vi "DAQ.Write.vi"(8 "error in (no error)":errorcluster, 10 "Write":T1, 11 "DAQmx.AO in":refnum<class "DAQmx.AO.lvclass">) -> (0 "error out":errorcluster, 2 "Written Waveform":waveform(dbl)[](array[waveform]), 3 "DAQmx.AO out":refnum<class "DAQmx.AO.lvclass">)   [LabVIEW 2016, in "DAQmx.AO.lvclass"]
uses:
  DAQmx.AO.lvclass
  C:/user/patrick/hg/levy_inst_lockin/src/SMOs/DAQmx/DAQmx.lvclass
  DAQ/Typedefs/PrivateEvents--DAQ.Write.ctl
  DAQmx/DAQmx.lvclass/DAQmx.ctl
  <vilib>/DAQmx/write.llb/DAQmx Write (Analog 1D Wfm NChan NSamp).vi
  <vilib>/DAQmx/miscellaneous.llb/DAQmx Fill In Error Info.vi
  <resource>/objmgr/daqmx.rc
  DAQmx/DAQmx.lvclass
  DAQ/DAQ.lvclass
panel:
  out "number of samples written per channel":u32
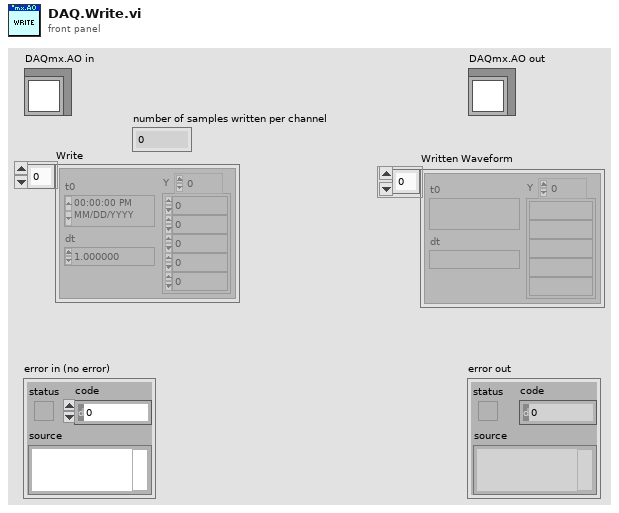
[diagram p1: front panel]
types:
  T1 = typedef "DAQ.lvclass/PrivateEvents--DAQ.Write.ctl" = waveform(dbl)[]
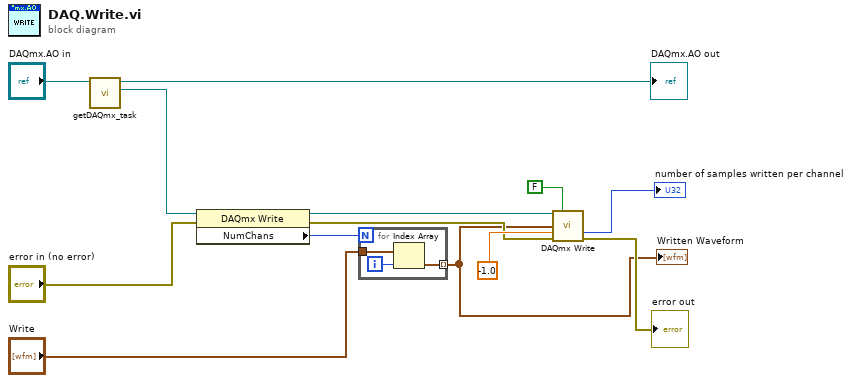
[diagram p0: block diagram]
diagram:
  n1 = call "getDAQmx_task.vi"("DAQmx in"="DAQmx.AO in") -> ("task"=w8:refnum<k21>, "DAQmx out"=→"DAQmx.AO out":refnum<class "DAQmx.AO.lvclass">)  [unwired: 8 in, 1 out]
  n2 = property class="DAQmx Write"(reference=w8, error in="error in (no error)") -> (reference out=w12:refnum<k21>, error out=w5:errorcluster, "NumChans"=w13:u32)
  n3 = for {
    N: w13 -> [_]
    tunnel: "Write" -> [w16]
    tunnel: [w15] -> w1 mode=indexing
    i -> [w14]
    n4 = Index Array(array=w16, index=w14) -> (element=w15:waveform(dbl))
  }
  "Written Waveform" <- w1
  n5 = call-poly <vilib>:"DAQmx Write.vi"("task/channels in"=w12, "auto start"=FALSE, "data"=w1, "timeout"=-1.0, "error in"=w5) -> ("number of samples written per channel"=→"number of samples written per channel":u32, "error out"=→"error out":errorcluster)  [unwired: 8 in, 1 out]
